vi "Robot Position Calculator.vi"(2 "Current wheel Angle":dbl, 3 "Wheel Encoder":dbl, 4 "Robot Angle Source":enum16{"Gyro", "Magnetometer", "Kalman Filter"}(ring)) -> (0 "Robot Y":dbl, 1 "Robot X":dbl)   [LabVIEW 2014]
uses:
  <vilib>/Rock Robotics/WPI/DriverStation/WPI_DriverStationRobotMode2.ctl
  Global Variables/Sensor Data (Edited).vi
  Global Variables/Settings.vi
  Global Variables/Miscalleneous.vi
  Robot Global Data.vi
panel:
  in  "Robot Length":dbl=27.5
  in  "Robot Width":dbl=28.0
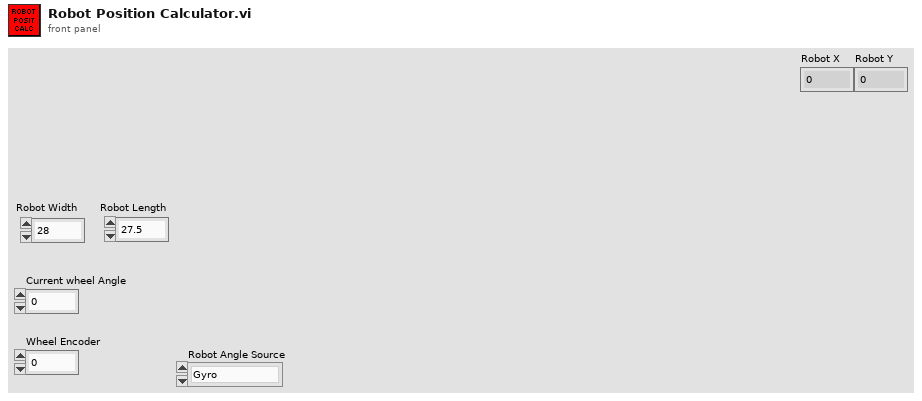
[diagram p1: front panel]
types:
  T1 = typedef "WPI_DriverStationRobotMode2.ctl" = enum16{"Autonomous Disabled", "Autonomous Enabled", "Teleop Disabled", "Teleop Enabled", "Disconnected", "Finish", "Test Disabled", "Test Enabled", "Emergency Stopped"}
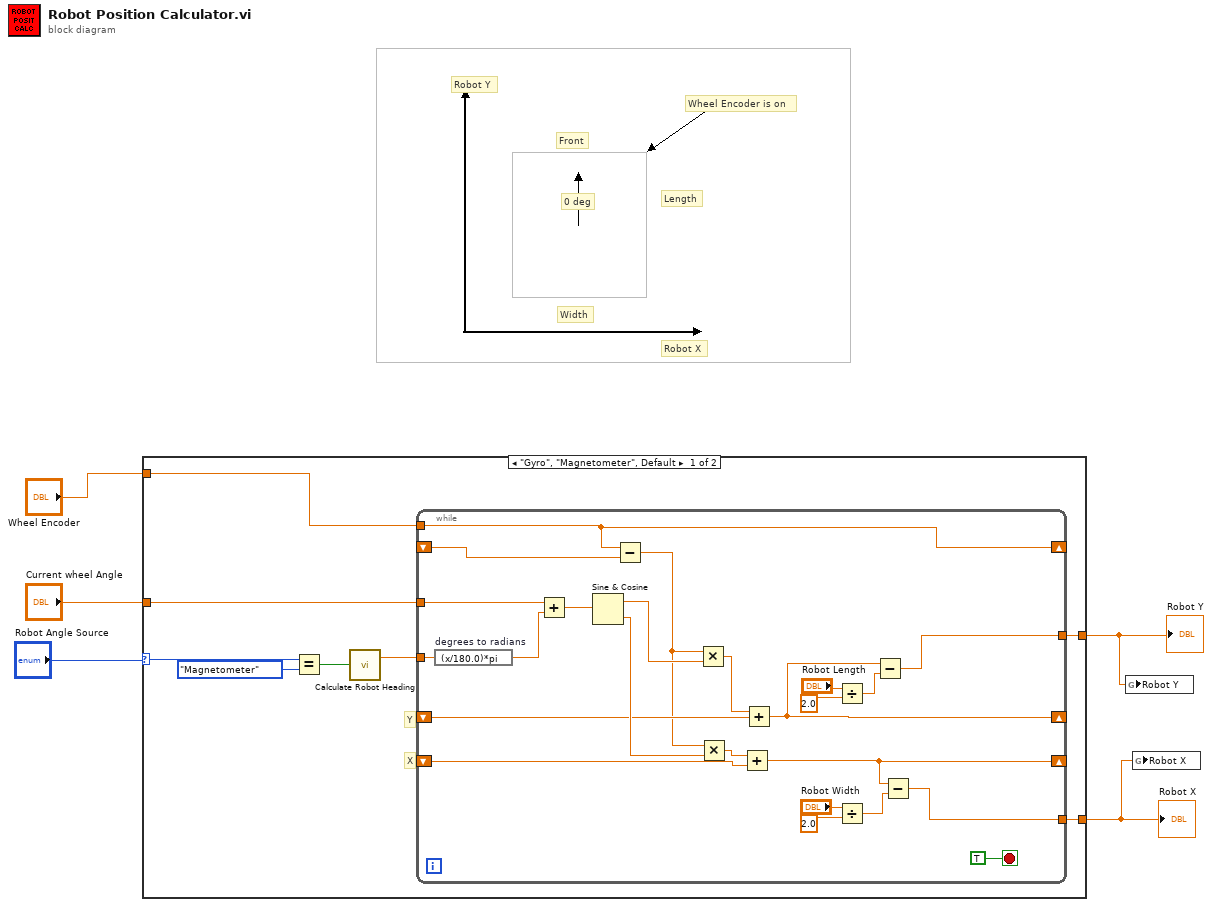
[diagram p0: block diagram]
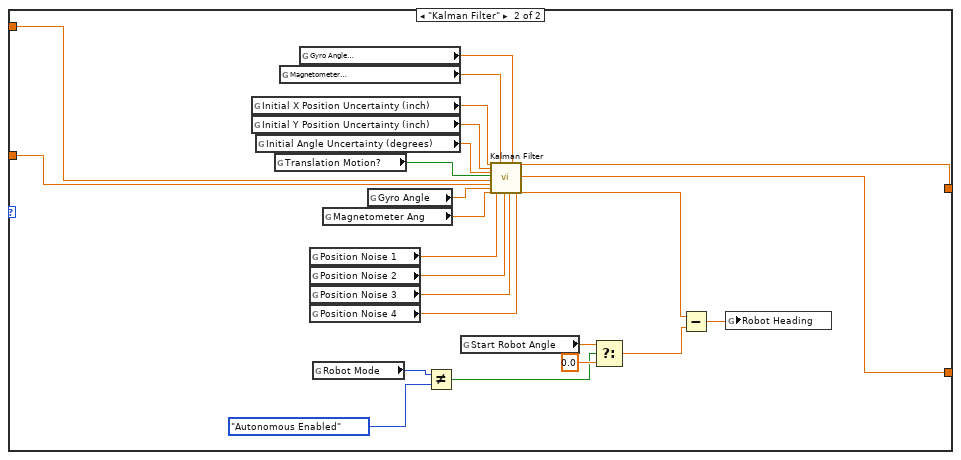
[diagram p2: hidden frame]
diagram:
  # "Wheel Encoder is on"
  # "Robot X"
  # "Robot Y"
  # "0 deg"
  # "Length"
  # "Front"
  # "Width"
  n1 = case shown="\"Gyro\", \"Magnetometer\", Default" "Robot Angle Source" {
    selector: "Robot Angle Source" -> [w9 _]
    tunnel: [w13 w47] -> w1
    tunnel: [w12 w46] -> w2
    tunnel: "Wheel Encoder" -> [w7 w58]
    tunnel: "Current wheel Angle" -> [w6 w61]
    frame "Gyro", "Magnetometer", Default {
      # "X"
      # "Y"
      n2 = Equal?(x=w9, y=enum16{"Gyro", "Magnetometer", "Kalman Filter"}."Magnetometer") -> (x = y?=w10:bool)
      n3 = call "Calculate Robot Heading.vi"("Magnetometer or Gyro used as Robot Angle? (Mag = T, Gyr = F)"=w10) -> ("Robot Angle"=w11:dbl)  [unwired: 3 in, 1 out]
      n4 = while {
        shift-right: [w15] -> _
        shift-left: _ -> [w23]
        shift-right: [w19] -> _
        shift-left: _ -> [w32]
        shift-right: [w26] -> _
        shift-left: _ -> [w33]
        tunnel: [w18] -> w13
        tunnel: [w24] -> w12
        tunnel: w11 -> [w16]
        tunnel: w7 -> [w15]
        tunnel: w6 -> [w14]
        stop <- TRUE stop-if-true
        n5 = expression code="(x/180.0)*pi" "degrees to radians"(w16) -> (w17:dbl)
        n6 = Add(x=w14, y=w17) -> (x+y=w21:dbl)
        n7 = Sine & Cosine(0:w21) -> (1:w36:dbl, 2:w35:dbl)
        n8 = Subtract(x=w15, y=w23) -> (x-y=w22:dbl)
        n9 = Multiply(x=w22, y=w36) -> (x*y=w31:dbl)
        n10 = Multiply(x=w22, y=w35) -> (x*y=w34:dbl)
        n11 = Add(x=w34, y=w33) -> (x+y=w26:dbl)
        n12 = Add(x=w31, y=w32) -> (x+y=w19:dbl)
        n13 = Divide(x="Robot Length", y=2.0) -> (x/y=w20:dbl)
        n14 = Divide(x="Robot Width", y=2.0) -> (x/y=w25:dbl)
        n15 = Subtract(x=w19, y=w20) -> (x-y=w18:dbl)
        n16 = Subtract(x=w26, y=w25) -> (x-y=w24:dbl)
      }
    }
    frame "Kalman Filter" {
      n17 = global read "Settings.vi" "Initial X Position Uncertainty (inch)"() -> (w57:dbl)
      n18 = global read "Settings.vi" "Initial Y Position Uncertainty (inch)"() -> (w56:dbl)
      n19 = global read "Settings.vi" "Initial Angle Uncertainty (degrees)"() -> (w55:dbl)
      n20 = global read "Miscalleneous.vi" "Translation Motion?"() -> (w54:bool)
      n21 = global read "Settings.vi" "Magnetometer\nStd. Deviation"() -> (w52:dbl)
      n22 = global read "Settings.vi" "Gyro Angle\nStd. Deviation"() -> (w53:dbl)
      n23 = global read "Settings.vi" "Position Noise 1"() -> (w51:dbl)
      n24 = global read "Settings.vi" "Position Noise 2"() -> (w50:dbl)
      n25 = global read "Settings.vi" "Position Noise 3"() -> (w48:dbl)
      n26 = global read "Settings.vi" "Position Noise 4"() -> (w49:dbl)
      n27 = global read "Robot Global Data.vi" "Robot Mode"() -> (w43:T1)
      n28 = global read "Sensor Data (Edited).vi" "Magnetometer Ang"() -> (w59:dbl)
      n29 = global read "Sensor Data (Edited).vi" "Gyro Angle"() -> (w60:dbl)
      n30 = Not Equal?(x=w43, y=WPI_DriverStationRobotMode2."Autonomous Enabled") -> (x != y?=w41:bool)
      n31 = global read "Miscalleneous.vi" "Start Robot Angle"() -> (w45:dbl)
      n32 = call "Kalman Filter.vi"("Initial X Position Uncertainty (inch)"=w57, "Initial Y Position Uncertainty (inch)"=w56, "Initial Angle Uncertainty (degrees)"=w55, "Translate\nMotion?"=w54, "Distance"=w58, "Wheel Angle"=w61, "Gyro Angle"=w60, "Magnetometer Angle"=w59, "Position Noise 1"=w51, "Magnetometer\nStd. Deviation"=w52, "Position Noise 2"=w50, "Position Noise 3"=w48, "Gyro Angle\nStd. Deviation"=w53, "Position Noise 4"=w49) -> ("Robot Position Y"=w47:dbl, "Robot Position X"=w46:dbl, "Robot Heading Angle"=w38:dbl)  [unwired: 11 in]
      n33 = Select(t=w45, s=w41, f=0.0) -> (s? t:f=w39:dbl)
      n34 = Subtract(x=w38, y=w39) -> (x-y=w40:dbl)
      n35 = global write "Sensor Data (Edited).vi" "Robot Heading"(w40) -> ()
    }
  }
  "Robot X" <- w2
  "Robot Y" <- w1
  n36 = global write "Sensor Data (Edited).vi" "Robot Y"(w1) -> ()
  n37 = global write "Sensor Data (Edited).vi" "Robot X"(w2) -> ()
